vi "Configure Reporting.vi"(8 "error in (no error)":errorcluster, 10 "Path":path, 11 "Execution API In":refnum<class "Execution API.lvclass">) -> (0 "error out":errorcluster, 3 "Execution API Out":refnum<class "Execution API.lvclass">)   [LabVIEW 2020, in "Execution API.lvclass"]
doc: "Configure reporting path and toggle automatic report generation."
uses:
  Execution API.lvclass
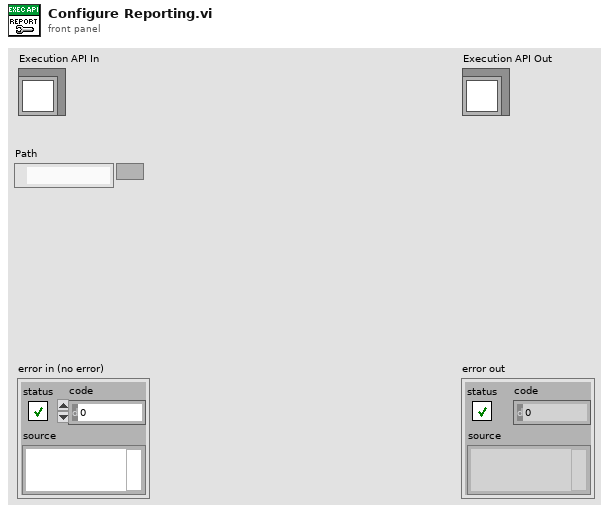
[diagram p1: front panel]
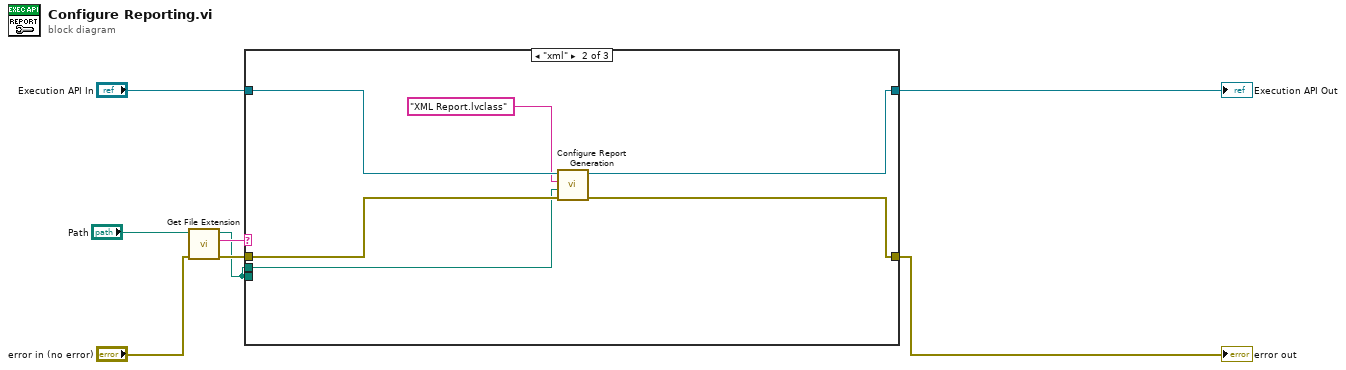
[diagram p0: block diagram]
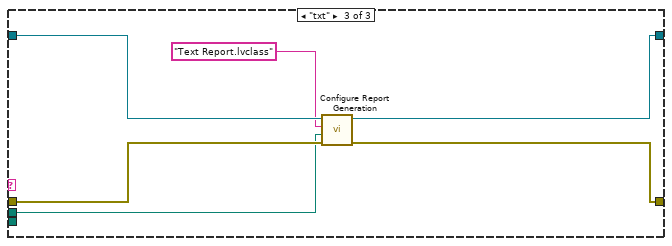
[diagram p3: hidden frame]
diagram:
  n1 = call <vilib>:"Get File Extension.vi"("error in (no error)"="error in (no error)", "file"="Path") -> ("error out"=w5:errorcluster, "lowercase file extension"=w7:string, "dup file"=w1:path)  [unwired: 5 in, 2 out]
  n2 = case shown="\"xml\"" w7 {
    tunnel: w5 -> [w9 w16 w22]
    tunnel: [w9 w13 w19] -> w4
    tunnel: [w10 w15 w21] -> w3
    tunnel: "Execution API In" -> [w10 w14 w20]
    tunnel: w1 -> [_ _ _]
    tunnel: w1 -> [_ w11 w17]
    frame Default {
    }
    frame "xml" {
      n3 = call "Configure Report Generation.vi"("error in (no error)"=w16, "Report File Path"=w11, "Report Type"="XML Report.lvclass" ("Plugin"), "Execution API in"=w14) -> ("error out"=w13:errorcluster, "Execution API out"=w15:refnum<class "Execution API.lvclass">)  [unwired: 6 in]
    }
    frame "txt" {
      n4 = call "Configure Report Generation.vi"("error in (no error)"=w22, "Report File Path"=w17, "Report Type"="Text Report.lvclass" ("Plugin"), "Execution API in"=w20) -> ("error out"=w19:errorcluster, "Execution API out"=w21:refnum<class "Execution API.lvclass">)  [unwired: 6 in]
    }
  }
  "error out" <- w4
  "Execution API Out" <- w3
